vi "fuzzy controler test.vi"() -> ()   [LabVIEW 2019]
uses:
  <vilib>/addons/Fuzzy Logic/TypeDefs/FL System.ctl
  <vilib>/addons/Fuzzy Logic/TypeDefs/FL Variable.ctl
  <vilib>/addons/Fuzzy Logic/TypeDefs/FL Membership Function.ctl
  <vilib>/addons/Fuzzy Logic/TypeDefs/FL Membership Function Shape.ctl
  <vilib>/addons/Fuzzy Logic/TypeDefs/FL Rule.ctl
  <vilib>/addons/Fuzzy Logic/TypeDefs/FL Antecedent.ctl
  <vilib>/addons/Fuzzy Logic/TypeDefs/FL Modifier.ctl
  <vilib>/addons/Fuzzy Logic/TypeDefs/FL Antecedent Connective.ctl
  <vilib>/addons/Fuzzy Logic/TypeDefs/FL Consequent.ctl
  <vilib>/addons/Fuzzy Logic/TypeDefs/FL Consequent Implication.ctl
  <vilib>/addons/Fuzzy Logic/TypeDefs/FL Defuzzification.ctl
  <vilib>/addons/Fuzzy Logic/TypeDefs/FL Interpolating polynomials.ctl
  <vilib>/addons/Fuzzy Logic/NI_Fuzzy_Logic_API.lvlib
  <vilib>/addons/Fuzzy Logic/FL Fuzzy Controller (MISO).vi
  <vilib>/measure/NI_MABase.lvlib
panel:
  in  "sampling info":cluster{"Fs":dbl, "#s":dbl}={"Fs"=1000.0, "#s"=1000.0} {"Fs" format="%.2p"}
  in  "reset signal":bool
  in  "duty cycle (%)":dbl=50.0 format="%0.2f"
  in  "amplitude":dbl=1.0 format="%0.2p"
  in  "frequency":dbl=10.0 format="%0.2p"
  out "Pulse Trend":waveform(dbl)[](graph) caption="Waveform Chart - Dark"
  out "appended array":string[](array[string])
  out "element":string
  out "Array":i32[](array[numeric])
  out "rules as text":string[](array[string])
  out "fuzzy system out":T1 {"user MF interpolating polynomials"."coa_x(y) coeff" format="%.4g"; "user MF interpolating polynomials"."Area(y) coeff" format="%.4g"; "user MF interpolating polynomials"."X(y) coeff" format="%.4g"; "user MF interpolating polynomials"."Y(x) coeff" format="%.4g"; "user MF interpolating polynomials"."Y" format="%.4g"; "user MF interpolating polynomials"."X" format="%.4g"; "defuzzification method" items=["Center of Area", "Modified Center of Area", "Center of Sums", "Center of Maximum", "Mean of Maximum"]; "rules"."consequents"."Var Index" min=0; "rules"."consequents"."Cond" items=["=", "!="]; "rules"."consequents"."MF Index" min=0; "rules"."antecedents"."Var Index" min=0; "rules"."antecedents"."Cond" items=["=", "!="]; "rules"."antecedents"."MF Index" min=0; "rules"."consequent implication" items=["Minimum", "Product"]; "rules"."antecedent connective" items=["AND (Minimum)", "AND (Product)", "OR (Maximum)", "OR (Probabilistic)"]; "output variables"."MFs"."shape" items=["Triangle", "Trapezoid", "Singleton", "Sigmoid", "Gaussian", "User-Defined"]; "input variables"."MFs"."shape" items=["Triangle", "Trapezoid", "Singleton", "Sigmoid", "Gaussian", "User-Defined"]}
  out "error out":errorcluster
  out "rule weights":dbl[](array[numeric])
  out "output value":dbl
  out "rule-invoked value?":bool
  in  "input values":dbl[](array[numeric])
  # "IF"
  # "THEN"
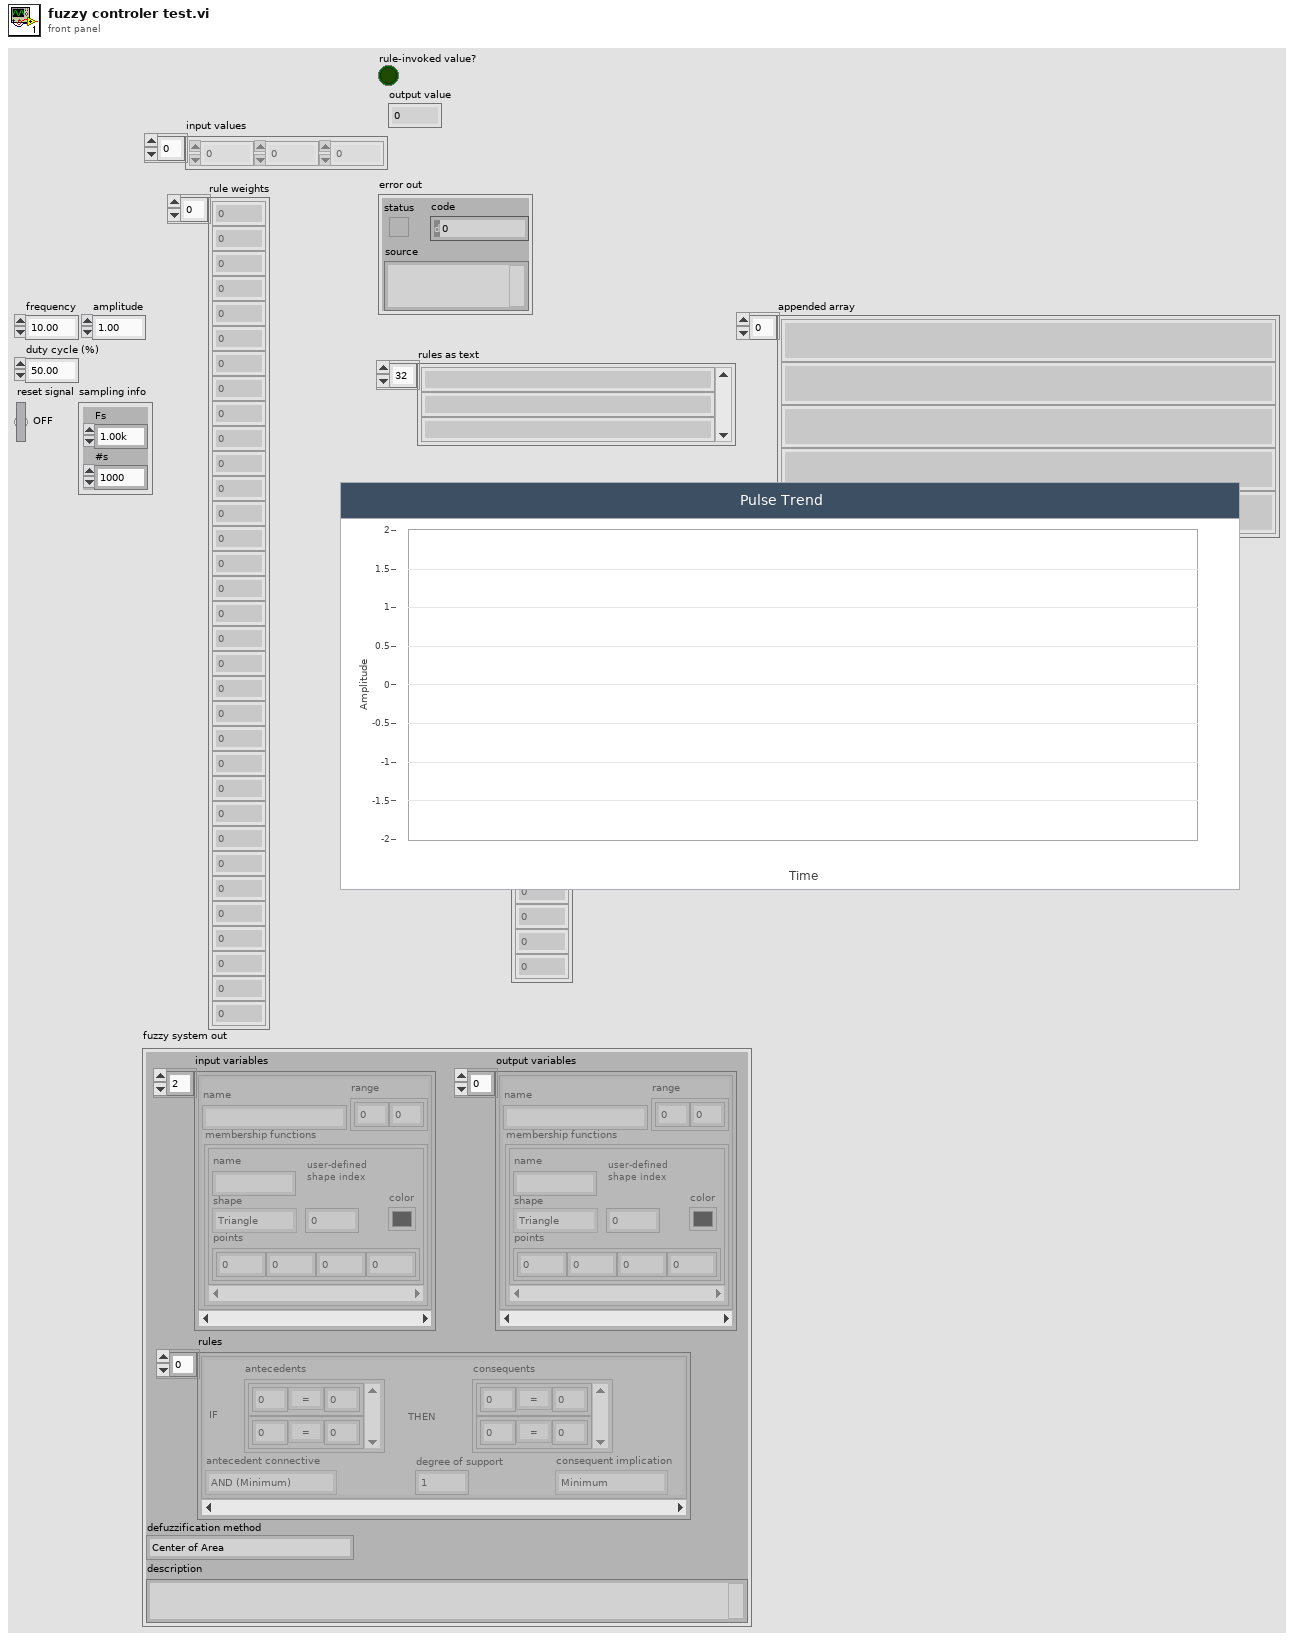
[diagram p1: front panel]
types:
  T1 = typedef "NI_Fuzzy_Logic_API.lvlib/FL System.ctl" = cluster{"input variables":T2[], "output variables":T2[], "rules":T5[], "defuzzification method":T11, "description":string, "user MF interpolating polynomials":T12[]}
  T2 = typedef "NI_Fuzzy_Logic_API.lvlib/FL Variable.ctl" = cluster{"name":string, "range":dbl[], "MFs":T3[]}
  T3 = typedef "NI_Fuzzy_Logic_API.lvlib/FL Membership Function.ctl" = cluster{"name":string, "shape":T4, "points":dbl[], "color":u32, "user-defined shape index":i32}
  T4 = typedef "NI_Fuzzy_Logic_API.lvlib/FL Membership Function Shape.ctl" = u16
  T5 = typedef "NI_Fuzzy_Logic_API.lvlib/FL Rule.ctl" = cluster{"antecedents":T6[], "antecedent connective":T8, "consequents":T9[], "consequent implication":T10, "degree of support":dbl}
  T6 = typedef "NI_Fuzzy_Logic_API.lvlib/FL Antecedent.ctl" = cluster{"Var Index":i32, "MF Index":i32, "Cond":T7}
  T7 = typedef "NI_Fuzzy_Logic_API.lvlib/FL Modifier.ctl" = u16
  T8 = typedef "NI_Fuzzy_Logic_API.lvlib/FL Antecedent Connective.ctl" = u16
  T9 = typedef "NI_Fuzzy_Logic_API.lvlib/FL Consequent.ctl" = cluster{"Var Index":i32, "MF Index":i32, "Cond":T7}
  T10 = typedef "NI_Fuzzy_Logic_API.lvlib/FL Consequent Implication.ctl" = u16
  T11 = typedef "NI_Fuzzy_Logic_API.lvlib/FL Defuzzification.ctl" = u16
  T12 = typedef "NI_Fuzzy_Logic_API.lvlib/FL Interpolating polynomials.ctl" = cluster{"X":dbl[], "Y":dbl[], "Y(x) coeff":dbl[][], "X(y) coeff":dbl[][], "Area(y) coeff":dbl[][], "coa_x(y) coeff":dbl[][]}
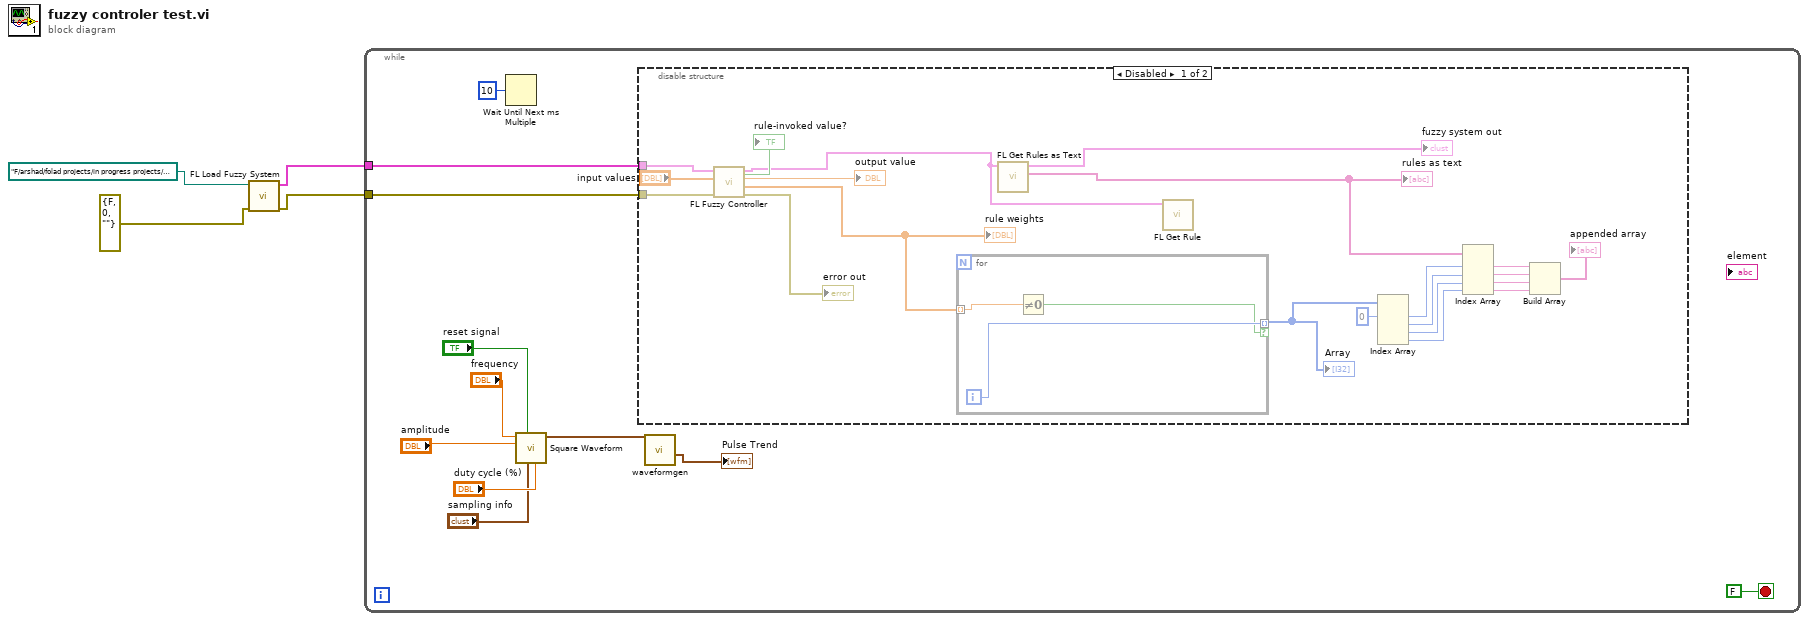
[diagram p0: block diagram]
diagram:
  n1 = call <vilib>:"FL Load Fuzzy System.vi"("error in (no error)"=errorcluster {"status"=FALSE, "code"=0, "source"=""}, "file path"=path "F:/arshad/folad projects/in progress projects/software/fuzzy1.fs") -> ("error out"=w1:errorcluster, "fuzzy system out"=w2:T1)  [unwired: 8 in]
  n2 = while {
    tunnel: w2 -> [w14]
    tunnel: w1 -> [w13]
    stop <- FALSE stop-if-true
    n3 = Wait Until Next ms Multiple(millisecond multiple=u32 10) -> ()  [unwired: 1 out]
    n4 = call <vilib>:"Square Waveform.vi"("duty cycle (%)"="duty cycle (%)", "sampling info"="sampling info", "reset signal"="reset signal", "amplitude"="amplitude", "frequency"="frequency") -> ("signal out"=w10:waveform(dbl))  [unwired: 5 in, 1 out]
    n5 = disable-structure shown="Disabled" {
      disable-tunnel: w14 -> [w32 _]
      disable-tunnel: w13 -> [w31 _]
      frame Disabled {
        n6 = call-poly <vilib>:"FL Fuzzy Controller.vi"("error in (no error)"=w31, "input values"="input values", "fuzzy system in"=w32) -> ("error out"=→"error out":errorcluster, "rule weights"=w28:dbl[], "output value"=→"output value":dbl, "fuzzy system out"=w29:T1, "rule-invoked value?"=→"rule-invoked value?":bool)  [unwired: 4 in]
        "rule weights" <- w28
        n7 = for {
          tunnel: w28 -> [w39] mode=indexing
          tunnel: [w38] -> w26 mode=indexing if=w37
          i -> [w38]
          n8 = Not Equal To 0?(x=w39) -> (x != 0?=w37:bool)
        }
        "Array" <- w26
        n9 = call <vilib>:"FL Get Rules as Text.vi"("fuzzy system in"=w29) -> ("rules as text"=w27:string[], "fuzzy system out"=→"fuzzy system out":T1)  [unwired: 8 in, 1 out]
        "rules as text" <- w27
        n10 = call <vilib>:"FL Get Rule.vi"("fuzzy system in"=w29) -> ()  [unwired: 4 in, 7 out]
        n11 = Index Array(array=w26, index #1=0 ("index")) -> (element #1=w24:i32, element #2=w23:i32, element #3=w22:i32, element #4=w21:i32)  [unwired: 3 in]
        n12 = Index Array(array=w27, index #1=w24, index #2=w23, index #3=w22, index #4=w21) -> (element #1=w20:string, element #2=w19:string, element #3=w18:string, element #4=w17:string)
        n13 = Build Array(w20, w19, w18, w17) -> (→"appended array":string[])
      }
      frame Enabled {
      }
    }
    n14 = call "waveformgen.vi"("trnd1"=w10) -> ("appended array"=→"Pulse Trend":waveform(dbl)[])  [unwired: 10 in]
  }
